vi "Choreo_Util_AllianceFlipX.vi"(11 "X":dbl) -> (3 "FlippedX":dbl)   [LabVIEW 2019, in "ChoreoLib.lvlib"]
doc: "trajectory, mirrored across the field midline.\n\nInputs: \n - ChoreoTrajectory - cluster - Input trajectory\n\nOutputs:\n - Flipped Trajectory - cluster - trajectory, mirrored across the field midline."
uses:
  ChoreoLib.lvlib
  Choreo_Choreo_Globals.vi
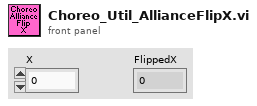
[diagram p1: front panel]
types:
  T1 = typedef "ChoreoLib.lvlib/Choreo_Util_AllianceFlipType.ctl" = enum16{"MIRRORED", "ROTATE_AROUND"}
  T2 = cluster{"Year":i32, "AllianceFlipType":T1, "FieldLength":dbl, "FieldWidth":dbl}
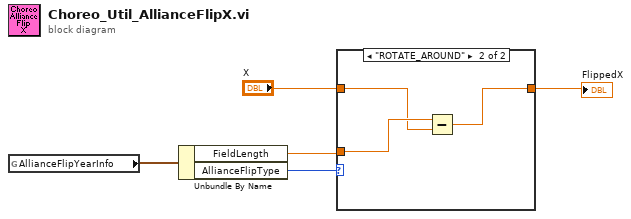
[diagram p0: block diagram]
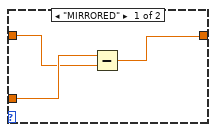
[diagram p2: hidden frame]
diagram:
  n1 = global read "Choreo_Choreo_Globals.vi" "AllianceFlipYearInfo"() -> (w5:T2)
  n2 = Unbundle By Name(w5) -> ("FieldLength"=w1:dbl, "AllianceFlipType"=w4:T1)
  n3 = case shown="\"ROTATE_AROUND\"" w4 {
    tunnel: "X" -> [w7 w10]
    tunnel: [w6 w9] -> w2
    tunnel: w1 -> [w8 w11]
    frame "MIRRORED" {
      n4 = Subtract(x=w8, y=w7) -> (x-y=w6:dbl)
    }
    frame "ROTATE_AROUND" {
      n5 = Subtract(x=w11, y=w10) -> (x-y=w9:dbl)
    }
  }
  "FlippedX" <- w2
